vi "String trim.vi"(8 "Auto":bool=TRUE, 9 "Repeat number":i32=1, 10 "Match string":string, 11 "Input string":string) -> (3 "Ouput string":string)   [LabVIEW 2018]
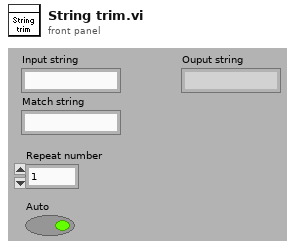
[diagram p1: front panel]
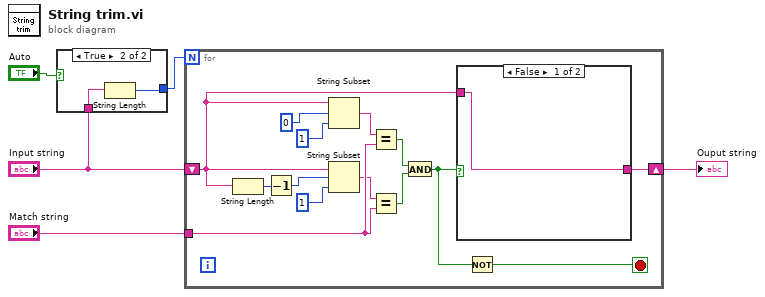
[diagram p0: block diagram]
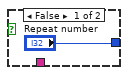
[diagram p2: hidden frame]
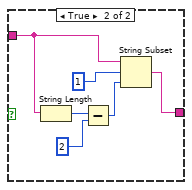
[diagram p3: hidden frame]
diagram:
  n1 = case shown="True" "Auto" {
    tunnel: ["Repeat number" w7] -> w3
    tunnel: "Input string" -> [_ w8]
    frame False {
    }
    frame True {
      n2 = String Length(string=w8) -> (length=w7:i32)
    }
  }
  n3 = for {
    N: w3 -> [_]
    tunnel: "Match string" -> [w22]
    shift-right: [w21] -> w4
    shift-left: "Input string" -> [w10]
    stop <- w9 stop-if-true
    n4 = String Length(string=w10) -> (length=w17:i32)
    n5 = Decrement(x=w17) -> (x-1=w11:i32)
    n6 = String Subset(string=w10, offset (0)=0 ("length (rest)"), length (rest)=1 ("length (rest)")) -> (substring=w16:string)
    n7 = String Subset(string=w10, offset (0)=w11, length (rest)=1 ("length (rest)")) -> (substring=w15:string)
    n8 = Equal?(x=w16, y=w22) -> (x = y?=w14:bool)
    n9 = Equal?(x=w15, y=w22) -> (x = y?=w13:bool)
    n10 = And(x=w14, y=w13) -> (x .and. y?=w12:bool)
    n11 = case shown="False" w12 {
      tunnel: w10 -> [w23 w25]
      tunnel: [w23 w24] -> w21
      frame False {
      }
      frame True {
        n12 = String Length(string=w25) -> (length=w28:i32)
        n13 = Subtract(x=w28, y=2) -> (x-y=w26:i32)
        n14 = String Subset(string=w25, offset (0)=1, length (rest)=w26) -> (substring=w24:string)
      }
    }
    n15 = Not(x=w12) -> (.not. x?=w9:bool)
  }
  "Ouput string" <- w4
